vi "3.4.vi"() -> ()   [LabVIEW 2017]
panel:
  out "字符串长度":dbl
  out "结果字符串":string
  in  "数值":dbl
  in  "尾":string
  in  "头":string
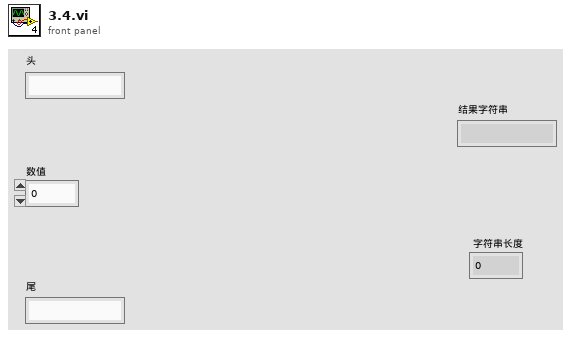
[diagram p1: front panel]
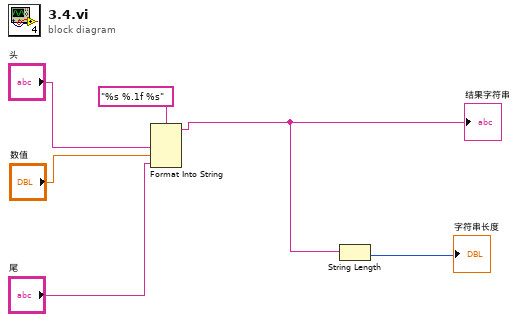
[diagram p0: block diagram]
diagram:
  n1 = Format Into String(format string="%s %.1f %s" ("格式字符串"), "头", "数值", "尾") -> (resulting string=w3:string)  [unwired: 2 in, 1 out]
  "结果字符串" <- w3
  n2 = String Length(string=w3) -> (length=→"字符串长度":i32)
